vi "^Swap_m.vi"(2 "^ Swap in":refnum<class "CtrlLine.lvclass">, 7 "QuWire in":refnum<class "QuWire.lvclass">, 13 "^ Ctrl in":refnum<class "CtrlLine.lvclass">) -> (8 "QuWire out":refnum<class "QuWire.lvclass">)   [LabVIEW 2020]
doc: "SWAP Gate (should be paired with an other qubit)\n\nExchanges the states of two qubits. \n\nMatrix: [[ 1, 0, 0, 0], [ 0, 0, 1, 0], [ 0, 1, 0, 0], [ 0, 0, 0, 1]]"
uses:
  QuSim/QuWire/QuWire.lvclass
  QuSim/QuWire/CtrlLine/CtrlLine.lvclass
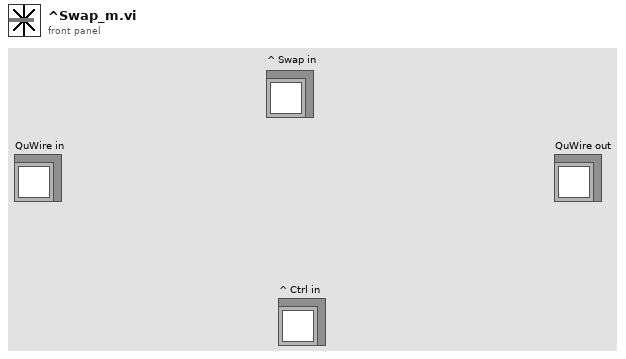
[diagram p1: front panel]
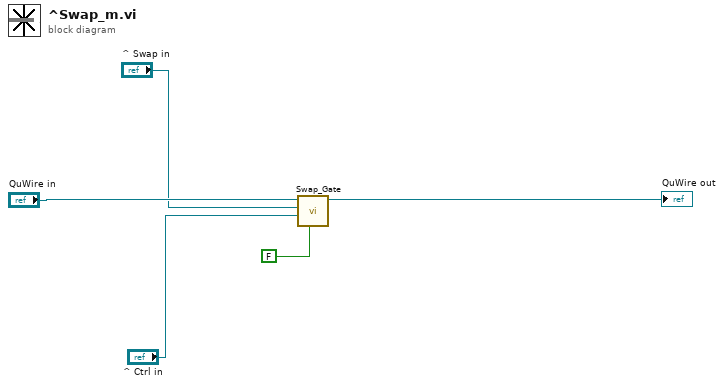
[diagram p0: block diagram]
diagram:
  n1 = call "Swap_Gate.vi"("Top Gate?"=FALSE, "d CtrlLine in"="^ Ctrl in", "u CtrlLine in"="^ Swap in", "QuWire in"="QuWire in") -> ("QuWire out"=→"QuWire out":refnum<class "QuWire.lvclass">)  [unwired: 5 in, 2 out]
